vi "temperature sub vi.vi"(9 "Boolean":bool, 11 "Slide":dbl) -> (3 "Numeric":dbl)   [LabVIEW 2018]
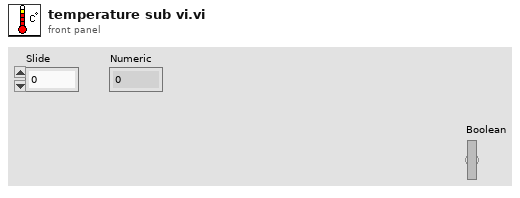
[diagram p1: front panel]
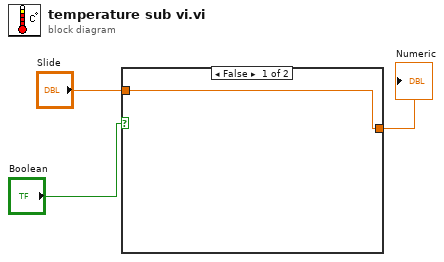
[diagram p0: block diagram]
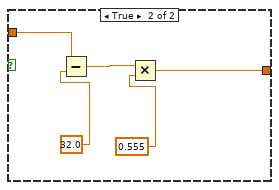
[diagram p2: hidden frame]
diagram:
  n1 = case shown="False" "Boolean" {
    tunnel: [w4 w9] -> w3
    tunnel: "Slide" -> [w4 w7]
    frame False {
    }
    frame True {
      n2 = Subtract(x=w7, y=32.0) -> (x-y=w8:dbl)
      n3 = Multiply(x=w8, y=0.555) -> (x*y=w9:dbl)
    }
  }
  "Numeric" <- w3
